vi "Test App Owned Process Context is Set.vi"(8 "error in (no error)":errorcluster, 11 "Application Test in":refnum<class "Application Test.lvclass">) -> (0 "error out":errorcluster, 3 "Application Test out":refnum<class "Application Test.lvclass">)   [LabVIEW 2020, in "Application Test.lvclass"]
uses:
  Application Test.lvclass
  Framework/Process/Process.lvclass
  Framework/Process/Process.lvclass/Process.ctl
  Framework/Application/Application.lvclass/Application.ctl
  <vilib>/Asteme/LUnit/Test Case.lvclass/Test Case.ctl
  <vilib>/Asteme/LUnit/LUnit Assertion Result.lvclass/LUnit Assertion Result.ctl
  Framework/Process/Protected/SubVIs/Set Context.vi
  Framework/Application/Private/Add Process to Map.vi
  Framework/Process/Protected/Messaging/Enqueue Message.vi
  Framework/Process/Public/Get Lifecycle State.vi
  Framework/Process/Protected/Messaging/Request Message.vi
  <vilib>/Asteme/LUnit/Palette/Fail.vi
  <vilib>/Asteme/LUnit/Palette/Pass.vi
  <vilib>/Asteme/LUnit/Set Assertion Type.vi
  Framework/Process/Private/SubVIs/Wait for finish.vi
  Framework/Process/Private/SubVIs/Set Lifecycle State.vi
  <vilib>/AdvancedString/1D String Array to Delimited String.vi
  <vilib>/Utility/error.llb/Clear Errors.vi
  Framework/Process/Private/SubVIs/Enqueue Request Message.vi
  <vilib>/Asteme/LUnit/Add test result.vi
  <vilib>/Asteme/LUnit/LUnit Write Passed.vi
  <vilib>/Asteme/LUnit/LUnit Get Test Case.vi
  <vilib>/Asteme/LUnit/LUnit Write Message.vi
  <vilib>/Asteme/LUnit/LUnit Write Description.vi
  <vilib>/Asteme/LUnit/LUnit Write Assertion Type.vi
  <vilib>/Asteme/LUnit/Read Test Case Name.vi
  Framework/Application/Application.lvclass
  C:/Users/anton/Documents/GitHub/Triarc-Framework/source/Framework/Process/Process.lvclass
  <vilib>/Utility/error.llb/Error Cluster From Error Code.vi
  Framework/Process/Private/SubVIs/Wait for Response Message.vi
  <vilib>/Asteme/LUnit/Assertion Result/LUnit Get Test Name.vi
  <vilib>/Asteme/LUnit/LUnit Assertion Result.lvclass
  C:/Users/anton/Documents/GitHub/Triarc-Framework/source/Framework/Base/Base.lvclass
  C:/Users/anton/Documents/GitHub/Triarc-Framework/source/Framework/Configuration File/Configuration File.lvclass
  C:/Users/anton/Documents/GitHub/Triarc-Framework/source/Framework/Application/Application.lvclass
  <vilib>/Asteme/LUnit/Test Case.lvclass
  C:/Users/anton/Documents/GitHub/Triarc-Framework/source/Framework Test/Process Test/Process Test.lvclass
  C:/Users/anton/Documents/GitHub/Triarc-Framework/source/Framework Test/Base Class Test/Base Class Test.lvclass
  C:/Program Files (x86)/National Instruments/LabVIEW 2020/vi.lib/Asteme/LUnit/Test Case.lvclass
  C:/Users/anton/Documents/GitHub/Triarc-Framework/source/Framework Test/Application Test/Application Test.lvclass
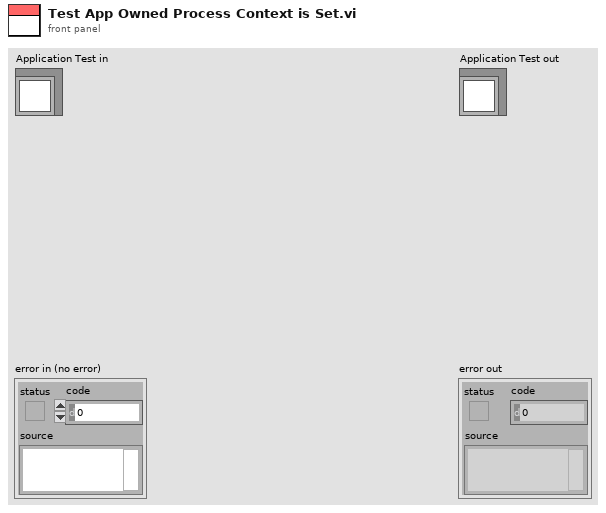
[diagram p1: front panel]
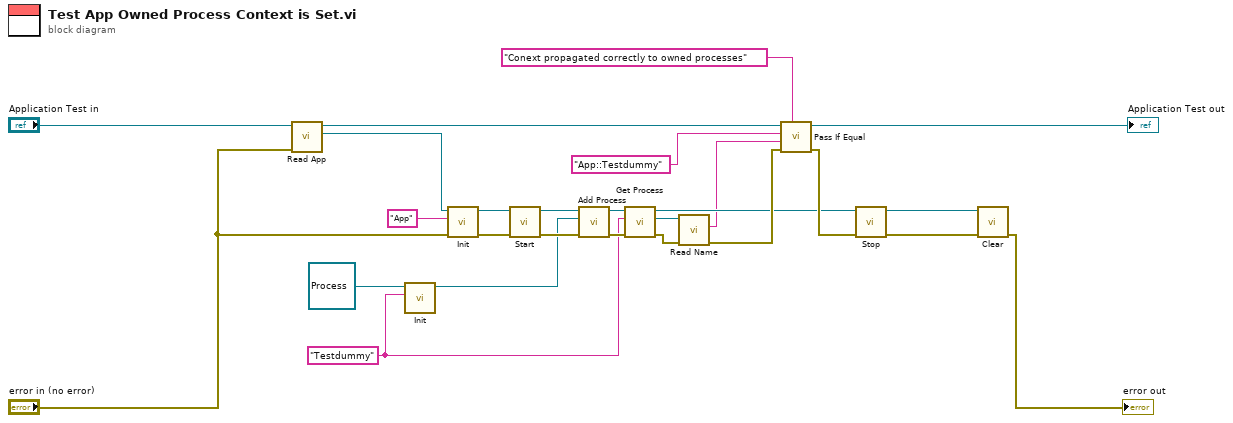
[diagram p0: block diagram]
diagram:
  w13 = "Testdummy" ("Name")
  n1 = call "Read App.vi"("error in (no error)"="error in (no error)", "Application Test In"="Application Test in") -> ("App out"=w25:refnum<class "Application.lvclass">, "Application Test Out"=w26:refnum<class "Application Test.lvclass">)  [unwired: 7 in, 1 out]
  n2 = call-dynamic "Init.vi"("Name"=w13, "Process In"=refnum<class "Process.lvclass"> refnum) -> ("Process Out"=w17:refnum<class "Process.lvclass">)  [unwired: 8 in, 1 out]
  n3 = call-dynamic "Init.vi"("error in (no error)"="error in (no error)", "Name"="App", "Process In"=w25) -> ("error out"=w23:errorcluster, "Process Out"=w24:refnum<class "Application.lvclass">)  [unwired: 7 in]
  n4 = call "Start.vi"("error in (no error)"=w23, "Process In"=w24) -> ("error out"=w20:errorcluster, "Process Out"=w11:refnum<class "Application.lvclass">)  [unwired: 8 in]
  n5 = call "Add Process.vi"("error in (no error)"=w20, "Process"=w17, "Rig In"=w11) -> ("error out"=w21:errorcluster, "Rig Out"=w4:refnum<class "Application.lvclass">)  [unwired: 7 in]
  n6 = call "Get Process.vi"("error in (no error)"=w21, "Process Name"=w13, "Rig In"=w4) -> ("error out"=w9:errorcluster, "App Process"=w10:refnum<class "Process.lvclass">, "Rig Out"=w7:refnum<class "Application.lvclass">)  [unwired: 6 in]
  n7 = call-dynamic "Read Name.vi"("error in (no error)"=w9, "Process In"=w10) -> ("error out"=w8:errorcluster, "Qualified Name"=w1:string)  [unwired: 6 in, 2 out]
  n8 = call <vilib>:"Pass If Equal.vi"("Description"="Conext propagated correctly to owned processes", "error in (no error)"=w8, "Actual"=w1, "Expected"="App::Testdummy", "Test Case In"=w26) -> ("error out"=w18:errorcluster, "Test Case Out"=→"Application Test out":refnum<class "Application Test.lvclass">)  [unwired: 5 in]
  n9 = call "Stop.vi"("error in (no error)"=w18, "Process In"=w7) -> ("error out"=w14:errorcluster, "Process Out"=w22:refnum<class "Application.lvclass">)  [unwired: 7 in, 1 out]
  n10 = call-dynamic "Clear.vi"("error in (no error)"=w14, "Application In"=w22) -> ("error out"=→"error out":errorcluster)  [unwired: 8 in, 1 out]
